vi "Read PROM.vi"(6 "I2C Slave Address":u8=119 format="%x", 7 "I2C Channel":u8, 8 "Error In":errorcluster, 11 "LINX Resource in":T1) -> (0 "Error Out":errorcluster, 1 "Correction Values":u16[](array[numeric]), 2 "Pass CRC?":bool, 3 "LINX Resource out":T1)   [LabVIEW 2014]
uses:
  <vilib>/MakerHub/LINX/Private/Type Defs/LINX Ref.ctl
  <vilib>/MakerHub/LINX/Private/Type Defs/Platform.ctl
  <vilib>/MakerHub/LINX/Private/Type Defs/Interface.ctl
  <vilib>/MakerHub/LINX/Private/Device/Type Defs/LINX Device Config.ctl
  <vilib>/MakerHub/LINX/Private/Device/Type Defs/TCP Config.ctl
  <vilib>/MakerHub/LINX/Private/Device/Type Defs/Channels.ctl
  <vilib>/MakerHub/LINX/Private/Local IO/LinxI2cWrite.vi
  <vilib>/MakerHub/LINX/Public/Utilities/Check Channel.vi
  <vilib>/MakerHub/LINX/Private/Utilties/Generate Error.vi
  <vilib>/MakerHub/LINX/LMH-LINX.lvlib
  <vilib>/MakerHub/LINX/Private/Device/Device.lvlib
panel:
  out "Address":i16[](array[numeric]) format="%x"
  # "Reserved"
  # "Coefficient 1"
  # "Coefficient 2"
  # "Coefficient 3"
  # "Coefficient 4"
  # "Coefficient 5"
  # "Coefficient 6"
  # "CRC"
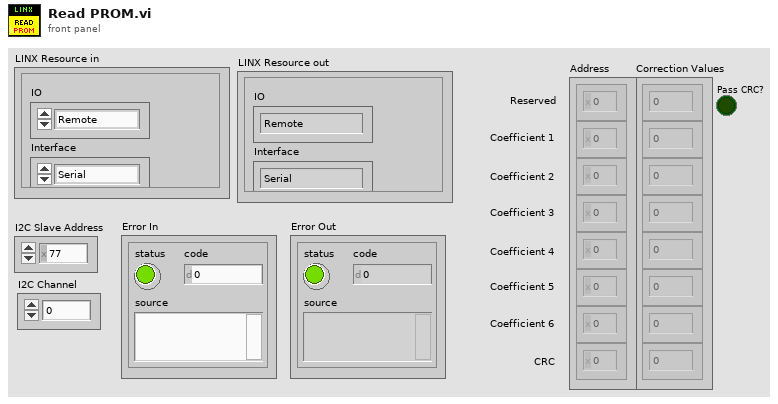
[diagram p1: front panel]
types:
  T1 = typedef "LMH-LINX.lvlib/LINX Ref.ctl" = cluster{"IO":T2, "Interface":T3, "LINX Device Config":T4}
  T2 = typedef "LMH-LINX.lvlib/Platform.ctl" = enum16{"Remote", "Local"}
  T3 = typedef "LMH-LINX.lvlib/Interface.ctl" = enum16{"Serial", "TCP"}
  T4 = typedef "LMH-LINX.lvlib/Device.lvlib/LINX Device Config.ctl" = cluster{"Interface":T3, "COM Port":refnum<visa-resource-name>, "TCP Configuration":T5, "Device Family":u8, "Device ID":u8, "Device Name":string, "TCP Ref":refnum<k5>, "Channels":T6}
  T5 = typedef "LMH-LINX.lvlib/Device.lvlib/TCP Config.ctl" = cluster{"IP Address":string, "Port":u16}
  T6 = typedef "LMH-LINX.lvlib/Channels.ctl" = cluster{"DI":u8[], "DO":u8[], "AI":u8[], "AO":u8[], "PWM":u8[], "QE":u8[], "UART":u8[], "I2C 2":u8[], "SPI":u8[], "CAN":u8[], "Servo":u8[], "AI Ref (V)":dbl, "AI Resolution (Bits)":u8, "AO Ref (V)":dbl, "AO Resolution (Bits)":u8}
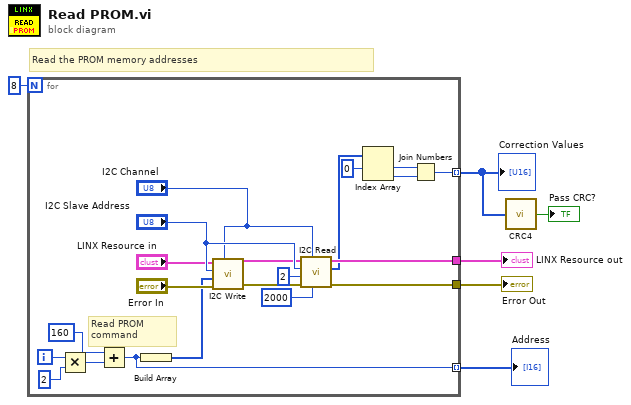
[diagram p0: block diagram]
diagram:
  # "Read the PROM memory addresses"
  n1 = for {
    N: 8 -> [_]
    tunnel: [w20] -> w5
    tunnel: [w19] -> w4
    tunnel: [w15] -> w2 mode=indexing
    tunnel: [w11] -> w3 mode=indexing
    i -> [w10]
    # "Read PROM command"
    n2 = Multiply(x=w10, y=2) -> (x*y=w8:i32)
    n3 = Add(x=u8 160, y=w8) -> (x+y=w11:i32)
    n4 = Build Array(w11) -> (w13:i32[])
    n5 = call <vilib>:"I2C Write.vi"("I2C Channel"="I2C Channel", "Error In"="Error In", "Data"=w13, "I2C Slave Address (0)"="I2C Slave Address", "LINX Resource"="LINX Resource in") -> ("Error Out"=w23:errorcluster, "LINX Resource"=w24:T1)  [unwired: 5 in]
    n6 = call <vilib>:"I2C Read.vi"("Timeout (1000 ms)"=u16 2000, "I2C Channel"="I2C Channel", "Error In"=w23, "Bytes To Read"=u8 2, "I2C Slave Address (0)"="I2C Slave Address", "LINX Resource"=w24) -> ("Error Out"=w19:errorcluster, "Data"=w18:u8[], "LINX Resource"=w20:T1)  [unwired: 3 in]
    n7 = Index Array(array=w18, index #1=0 ("index")) -> (element #1=w17:u8, element #2=w16:u8)  [unwired: 1 in]
    n8 = Join Numbers(hi=w17, lo=w16) -> ((hi.lo)=w15:u16)
  }
  "LINX Resource out" <- w5
  "Error Out" <- w4
  "Correction Values" <- w2
  "Address" <- w3
  n9 = call "CRC4.vi"("Correction Values"=w2) -> ("Pass CRC?"=→"Pass CRC?":bool)  [unwired: 4 in]
